vi "Test save scan.vi"(10 "Scan parameter":T1={"Horizontal axis"=enum."x", "Vertical axis"=enum."y", "vertical num"=100, "vertical end"=50.0, "vertical start"=40.0, "horizontal num"=100, "horizontal end"=25.0, "horizontal start"=15.0}) -> (3 "tdms file out":refnum<k34>)   [LabVIEW 2020]
uses:
  Labview Library/Libraries/Basic Experiment/Scan Settings.ctl
  Axis Enum.ctl
  Labview Library/Libraries/LaoJi/UT_Utilities/Utilities.lvlib
  Labview Library/Libraries/Basic Experiment/Basic Experiment.lvlib
panel:
  in  "file path":path=path "G:/Default/Save/demo Save_Y2021_M12_D01_21_20_53.tdms"
  out "Array":dbl[](array[numeric])=[0.0, 1.0]
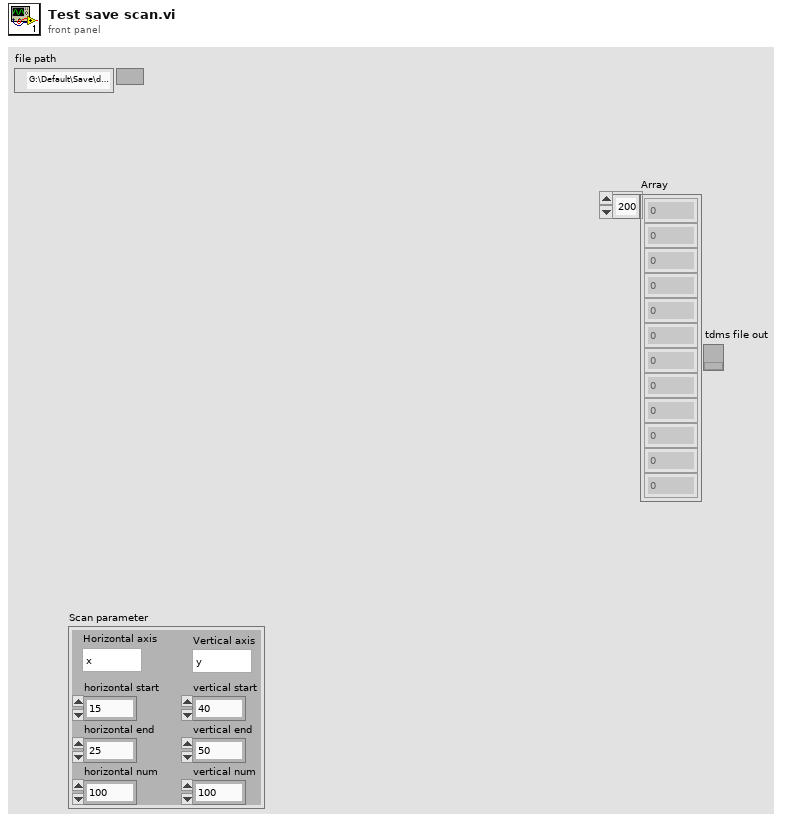
[diagram p1: front panel]
types:
  T1 = typedef "Basic Experiment.lvlib/Scan Settings.ctl" = cluster{"Horizontal axis":T2, "Vertical axis":T2, "vertical num":u32, "vertical end":dbl, "vertical start":dbl, "horizontal num":u32, "horizontal end":dbl, "horizontal start":dbl}
  T2 = typedef "Axis Enum.ctl" = enum16{"x", "y", "z"}
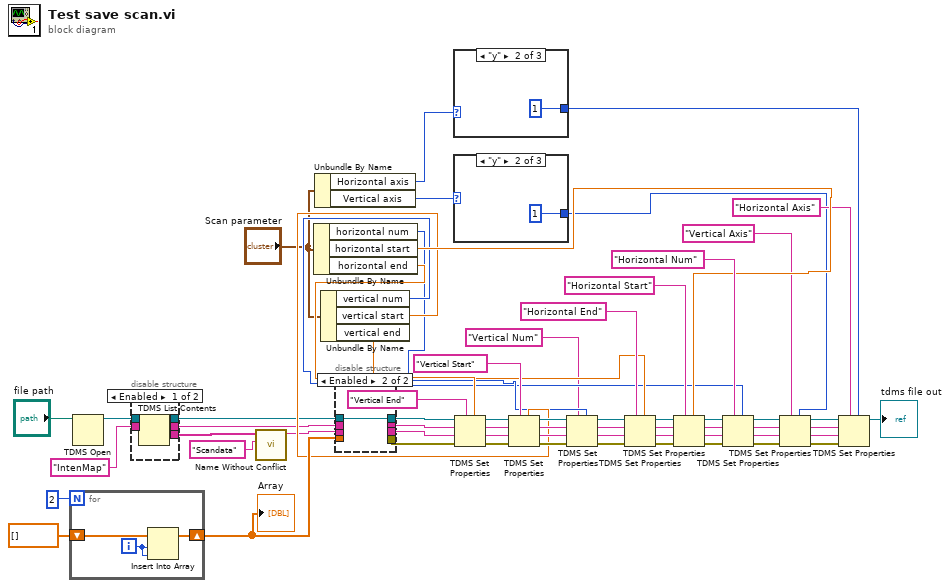
[diagram p0: block diagram]
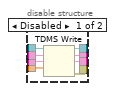
[diagram p3: hidden frame]
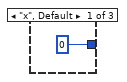
[diagram p4: hidden frame]
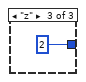
[diagram p5: hidden frame]
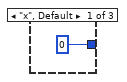
[diagram p6: hidden frame]
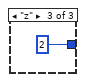
[diagram p7: hidden frame]
diagram:
  n1 = for {
    N: 2 -> [_]
    shift-right: [w66] -> w62
    shift-left: dbl[] [] -> [w65]
    i -> [w64]
    n2 = Insert Into Array(array=w65, index=w64, new element=w64) -> (w66:dbl[])
  }
  "Array" <- w62
  n3 = TDMS Open(11:"file path") -> (3:w1:refnum<k34>)  [unwired: 6 in, 1 out]
  n4 = disable-structure shown="Enabled" {
    disable-tunnel: [w71 w72] -> w5
    disable-tunnel: [w70 _] -> w4
    disable-tunnel: [w69 _] -> w3
    disable-tunnel: "IntenMap" ("group name in (Untitled)") -> [w68 _]
    disable-tunnel: w1 -> [w67 w72]
    frame Enabled {
      n5 = TDMS List Contents(6:w68, 7:w67) -> (1:w69:string[], 2:w70:string, 3:w71:refnum<k34>)  [unwired: 1 in, 1 out]
    }
    frame Disabled {
    }
  }
  n6 = call "Name Without Conflict.vi"("name"="Scandata", "Exist Name Array"=w3) -> ("New Name"=w9:string)  [unwired: 9 in]
  n7 = Unbundle By Name("Scan parameter") -> ("horizontal num"=w33:u32, "horizontal start"=w39:dbl, "horizontal end"=w34:dbl)
  n8 = Unbundle By Name("Scan parameter") -> ("Horizontal axis"=w14:T2, "Vertical axis"=w13:T2)
  n9 = Unbundle By Name("Scan parameter") -> ("vertical num"=w35:u32, "vertical start"=w37:dbl, "vertical end"=w36:dbl)
  n10 = disable-structure shown="Enabled" {
    disable-tunnel: w62 -> [w80 _]
    disable-tunnel: [w79 _] -> w61
    disable-tunnel: [w78 w81] -> w60
    disable-tunnel: [w77 _] -> w38
    disable-tunnel: w9 -> [w76 _]
    disable-tunnel: [w75 _] -> w8
    disable-tunnel: w5 -> [w74 w81]
    disable-tunnel: w4 -> [w73 _]
    frame Disabled {
      n11 = TDMS Write(0:w74, 5:w73, 7:w76, 9:w80) -> (4:w78:refnum<k34>, 6:w79:string, 8:w75:string, 15:w77:errorcluster)  [unwired: 2 in]
    }
    frame Enabled {
    }
  }
  n12 = case shown="\"y\"" w14 {
    tunnel: [0 1 2] -> w12
    frame "x", Default {
    }
    frame "y" {
    }
    frame "z" {
    }
  }
  n13 = case shown="\"y\"" w13 {
    tunnel: [0 1 2] -> w11
    frame "x", Default {
    }
    frame "y" {
    }
    frame "z" {
    }
  }
  n14 = TDMS Set Properties(5:w36, 7:"Vertical End" ("group name in (Untitled)"), 8:w38, 9:w8, 10:w61, 11:w60) -> (0:w59:errorcluster, 1:w58:string, 2:w57:string, 3:w56:refnum<k34>)
  n15 = TDMS Set Properties(5:w37, 7:"Vertical Start" ("group name in (Untitled)"), 8:w59, 9:w58, 10:w57, 11:w56) -> (0:w54:errorcluster, 1:w53:string, 2:w52:string, 3:w51:refnum<k34>)
  n16 = TDMS Set Properties(5:w35, 7:"Vertical Num" ("group name in (Untitled)"), 8:w54, 9:w53, 10:w52, 11:w51) -> (0:w43:errorcluster, 1:w44:string, 2:w45:string, 3:w46:refnum<k34>)
  n17 = TDMS Set Properties(5:w34, 7:"Horizontal End" ("group name in (Untitled)"), 8:w43, 9:w44, 10:w45, 11:w46) -> (0:w47:errorcluster, 1:w48:string, 2:w16:string, 3:w17:refnum<k34>)
  n18 = TDMS Set Properties(5:w39, 7:"Horizontal Start" ("group name in (Untitled)"), 8:w47, 9:w48, 10:w16, 11:w17) -> (0:w49:errorcluster, 1:w50:string, 2:w15:string, 3:w18:refnum<k34>)
  n19 = TDMS Set Properties(5:w33, 7:"Horizontal Num" ("group name in (Untitled)"), 8:w49, 9:w50, 10:w15, 11:w18) -> (0:w30:errorcluster, 1:w29:string, 2:w28:string, 3:w27:refnum<k34>)
  n20 = TDMS Set Properties(5:w11, 7:"Vertical Axis" ("group name in (Untitled)"), 8:w30, 9:w29, 10:w28, 11:w27) -> (0:w26:errorcluster, 1:w25:string, 2:w24:string, 3:w23:refnum<k34>)
  n21 = TDMS Set Properties(5:w12, 7:"Horizontal Axis" ("group name in (Untitled)"), 8:w26, 9:w25, 10:w24, 11:w23) -> (3:→"tdms file out":refnum<k34>)  [unwired: 3 out]
